vi "SmartMotor_SendMoveCmd - Position Move - single motor - v2.vi"(6 "ReadWait":u32=50, 7 "MotorSpecifier(M1)":T1=enum."M1", 8 "error in (no error)":errorcluster, 9 "posType":T2=enum."Relative" caption="position type (Relative)", 10 "Displacement (cnts)":dbl, 11 "VISA Ref":refnum<visa-resource-name>) -> (0 "error out":errorcluster, 2 "Cmd Str out":string, 3 "VISA Out":refnum<visa-resource-name>)   [LabVIEW 2017]
doc: "Developed by Kevin Thompson\nkevin@thompsonengineering.net\n\nCopyright 2018-2020\nThompson Engineering, LLC"
uses:
  TD PositionType_enum.ctl
  TD SerialBusMotorSpecifier_enum.ctl
  TD MotorCommands - single motor--enum.ctl
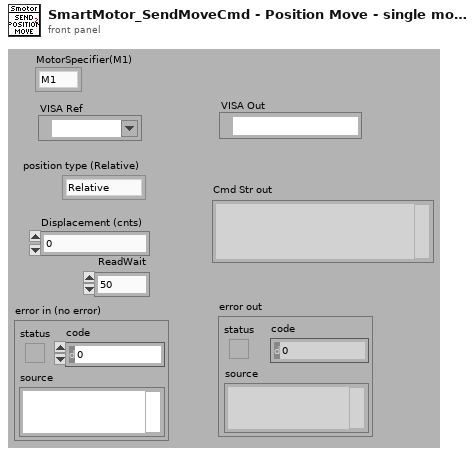
[diagram p1: front panel]
types:
  T1 = typedef "TD SerialBusMotorSpecifier_enum.ctl" = enum16{"None", "Global", "M1", "M2", "M3"}
  T2 = typedef "TD PositionType_enum.ctl" = enum16{"Absolute", "Relative"}
  T3 = typedef "TD MotorCommands - single motor--enum.ctl" = enum16{"Unlisted", "AbortMotion", "StopMotion", "DisableMotor", "ClearErrors", "ZeroEncoder", "SetMode", "GO", "SetEncoder", "En/Ds LmtSwitchs"}
  T4 = cluster{"String Input":string, "ExpectResponse":bool}
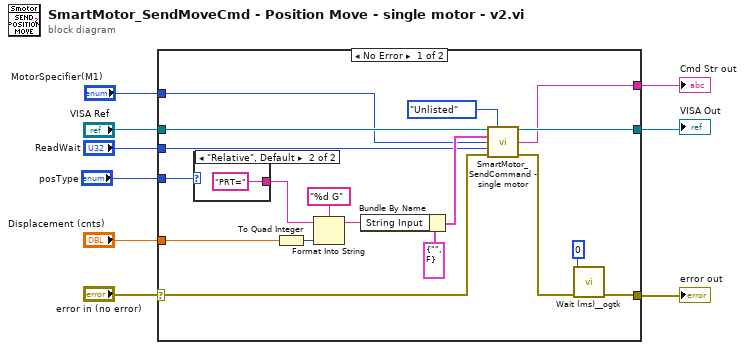
[diagram p0: block diagram]
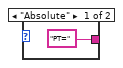
[diagram p2: hidden frame]
diagram:
  n1 = case shown="No Error" "error in (no error)" {
    selector: "error in (no error)" -> [w26 w31]
    tunnel: [w14 _] -> w9
    tunnel: "VISA Ref" -> [w27 w30]
    tunnel: [w24 w31] -> w7
    tunnel: [w15 w30] -> w5
    tunnel: "Displacement (cnts)" -> [w18 _]
    tunnel: "posType" -> [w13 _]
    tunnel: "ReadWait" -> [w11 _]
    tunnel: "MotorSpecifier(M1)" -> [w10 _]
    frame No Error {
      n2 = case shown="\"Relative\", Default" w13 {
        tunnel: ["PT=" "PRT="] -> w12
        frame "Absolute" {
        }
        frame "Relative", Default {
        }
      }
      n3 = To Quad Integer(1:w18) -> (0:w25:i64)
      n4 = Format Into String(format string="%d G", initial string=w12, w25) -> (resulting string=w21:string)  [unwired: 1 in, 1 out]
      n5 = Bundle By Name(cluster=T4 {"String Input"="", "ExpectResponse"=FALSE} ("Adhoc Input"), "String Input"=w21) -> (w22:T4)
      n6 = call "SmartMotor_SendCommand - single motor.vi"("VISA In"=w27, "MotorCmd"=TD_MotorCommands_-_single_motor--enum."Unlisted", "Adhoc Input"=w22, "MotorSpecifier(M1)"=w10, "ReadWait"=w11, "error in"=w26) -> ("VISA Out"=w15:refnum<visa-resource-name>, "Cmd Str out"=w14:string, "error out"=w16:errorcluster)  [unwired: 6 in, 1 out]
      n7 = call <userlib>:"Wait (ms)__ogtk.vi"("error in (no error)"=w16, "milliseconds to wait"=u32 0 ("wait (ms)")) -> ("error out"=w24:errorcluster)  [unwired: 8 in, 1 out]
    }
    frame Error {
    }
  }
  "error out" <- w7
  "Cmd Str out" <- w9
  "VISA Out" <- w5
